vi "HFRR ADV v01.vi"() -> ()   [LabVIEW 2025] (continued)
              tunnel: w635 -> [w689 _]
              frame False {
                n427 = Equal?(x=w692, y="\"line\"") -> (x = y?=w694:bool)
                n428 = case shown="True" w694 {
                  tunnel: w693 -> [_ w709]
                  tunnel: w691 -> [w696 w708]
                  tunnel: [w696 w706] -> w690
                  tunnel: w689 -> [_ w705]
                  frame False {
                  }
                  frame True {
                    w704 = 0.0 ("Major Axis")
                    n429 = Match Pattern(string=w709, regular expression="\"length_px\":") -> (after substring=w707:string)  [unwired: 1 in, 3 out]
                    n430 = property on="Major Axis" class="DigNum (strict)"("Caption.Text"="") -> ()  [unwired: 2 in, 2 out]
                    n431 = property on="Minor Axis" class="DigNum (strict)"("Caption.Text"="") -> ()  [unwired: 2 in, 2 out]
                    n432 = property on="Average" class="DigNum (strict)"("Caption.Text"="Line") -> ()  [unwired: 2 in, 2 out]
                    n433 = Fract/Exp String To Number(string=w707, default (0 dbl)=0.0 ("default (0 DBL)")) -> (number=w703:dbl)  [unwired: 2 in, 1 out]
                    "Pixel Value" <- w703
                    n434 = Multiply(x=w703, y=w705) -> (x*y=w716:dbl)
                    n435 = Multiply(x=w716, y=1000.0) -> (x*y=w699:dbl)
                    n436 = Divide(x=w699, y=1000.0) -> (x/y=w702:dbl)
                    n437 = local write "Measurment (mm)"(w702) -> ()
                    n438 = Bundle By Name(cluster=w708, "average"=w699) -> (w706:cluster{"major":dbl, "minor":dbl, "average":dbl})
                    n439 = Number To Fractional String(number=w699, precision (6)=i16 1) -> (F-format string=w698:string)  [unwired: 2 in]
                    n440 = local write "Minor Axis"(w704) -> ()
                    n441 = local write "Major Axis"(w704) -> ()
                    n442 = Fract/Exp String To Number(string=w698) -> (number=w697:dbl)  [unwired: 3 in, 1 out]
                    n443 = local write "Average"(w697) -> ()
                  }
                }
              }
              frame True {
                w736 = 1000.0 ("y")
                w742 = 0.0 ("default (0 DBL)")
                n444 = Match Pattern(string=w748, regular expression=" \"width_px\":") -> (after substring=w746:string)  [unwired: 1 in, 3 out]
                n445 = Match Pattern(string=w746, regular expression="\"height_px\":") -> (before substring=w744:string, after substring=w743:string)  [unwired: 1 in, 2 out]
                n446 = Fract/Exp String To Number(string=w744, default (0 dbl)=w742) -> (number=w741:dbl)  [unwired: 2 in, 1 out]
                n447 = Fract/Exp String To Number(string=w743, default (0 dbl)=w742) -> (number=w740:dbl)  [unwired: 2 in, 1 out]
                n448 = Multiply(x=w741, y=w739) -> (x*y=w738:dbl)
                n449 = Multiply(x=w740, y=w739) -> (x*y=w737:dbl)
                n450 = Multiply(x=w738, y=w736) -> (x*y=w722:dbl)
                n451 = Multiply(x=w737, y=w736) -> (x*y=w720:dbl)
                n452 = Add(x=w722, y=w720) -> (x+y=w734:dbl)
                n453 = property on="Major Axis" class="DigNum (strict)"("Caption.Text"="Major Axis") -> ()  [unwired: 2 in, 2 out]
                n454 = property on="Minor Axis" class="DigNum (strict)"("Caption.Text"="Minor Axis") -> ()  [unwired: 2 in, 2 out]
                n455 = property on="Average" class="DigNum (strict)"("Caption.Text"="Average") -> ()  [unwired: 2 in, 2 out]
                n456 = Divide(x=w734, y=2.0) -> (x/y=w718:dbl)
                n457 = Bundle By Name(cluster=w735, "major"=w722, "minor"=w720, "average"=w718) -> (w732:cluster{"major":dbl, "minor":dbl, "average":dbl})
                n458 = Number To Fractional String(number=w720, precision (6)=i16 1) -> (F-format string=w727:string)  [unwired: 2 in]
                n459 = Number To Fractional String(number=w718, precision (6)=i16 1) -> (F-format string=w728:string)  [unwired: 2 in]
                n460 = Number To Fractional String(number=w722, precision (6)=i16 1) -> (F-format string=w726:string)  [unwired: 2 in]
                n461 = Fract/Exp String To Number(string=w727) -> (number=w719:dbl)  [unwired: 3 in, 1 out]
                n462 = Fract/Exp String To Number(string=w728) -> (number=w717:dbl)  [unwired: 3 in, 1 out]
                n463 = Fract/Exp String To Number(string=w726) -> (number=w721:dbl)  [unwired: 3 in, 1 out]
                n464 = local write "Major Axis"(w721) -> ()
                n465 = local write "Average"(w717) -> ()
                n466 = local write "Minor Axis"(w719) -> ()
              }
            }
            n467 = case shown="\"Measrument\", Default" w631 {
              tunnel: w634 -> [w661 _]
              tunnel: w633 -> [w660 _]
              tunnel: [w657 w686] -> w632
              tunnel: w630 -> [w659 w686]
              tunnel: w629 -> [w658 _]
              tunnel: w626 -> [w656 _]
              frame "Measrument", Default {
                n468 = stacked-sequence {
                  tunnel: w661 -> [w679 _]
                  tunnel: w660 -> [w677 _]
                  tunnel: w659 -> [w675 _]
                  tunnel: w658 -> [w674 _]
                  tunnel: [w669 _] -> w657
                  tunnel: w656 -> [w662 _]
                  frame #0 {
                    n469 = call "IMAGE ANALYSIS.vi"("Enum"=POST_ANALYSIS_ENUM."SAVE IMAGE", "error in"=w675, "IMAGE FILE PATH"=w674) -> ("error out"=w673:errorcluster)  [unwired: 7 in, 1 out]
                    n470 = call "Stall Data Flow.vim"("value in"=w673, "milliseconds to wait"=u32 1000) -> ("value out"=w664:errorcluster)  [unwired: 1 out]
                    n471 = local read "Test File List :"() -> (w681:string)
                    n472 = call "IMAGE ANALYSIS.vi"("Enum"=POST_ANALYSIS_ENUM."MINIMIZE UI", "error in"=w664) -> ("error out"=w671:errorcluster)  [unwired: 8 in, 1 out]
                    n473 = Bundle By Name(cluster=T20 {"File Name"="", "Test Method"="", "Operator"="", "Fuel Description"="", "Date and time"=""} ("Main Ref"), "Test Method"=w662, "File Name"=w681) -> (w682:T20)
                    n474 = call "Stall Data Flow.vim"("value in"=w671, "milliseconds to wait"=u32 1500) -> ("value out"=w666:errorcluster)  [unwired: 1 out]
                    n475 = call "duf file read.vi"("error in (no error)"=w666, "Main Ref"=w682) -> ("error out"=w680:errorcluster, "Main Ref 2"=w678:T20)  [unwired: 8 in]
                    n476 = call "DETECTION REPORT for manual.vi"("error in (no error)"=w680, "return value 3"=w677, "Image File Path"=w679, "Main Ref"=w678) -> ("error out"=w676:errorcluster)  [unwired: 7 in]
                    n477 = call <vilib>:"Clear Errors.vi"("error in (no error)"=w676) -> ("error out"=w667:errorcluster)  [unwired: 5 in, 1 out]
                    n478 = call "IMAGE ANALYSIS.vi"("Enum"=POST_ANALYSIS_ENUM."MINIMIZE UI", "error in"=w667) -> ("error out"=w669:errorcluster)  [unwired: 8 in, 1 out]
                  }
                  frame #1 {
                    n479 = local write "Main Tab"(T2."HOME" ("Main Tab")) -> ()
                    n480 = local write "Main Dashboard Buttons"(T1."Home" ("Main Dashboard Buttons")) -> ()
                  }
                }
              }
              frame "Calibrate" {
              }
            }
          }
          frame #2 {
            n481 = Not(x=w751) -> (.not. x?=w750:bool)
            n482 = local write "Confirm Measrurement"(w750) -> ()
            n483 = local read "Calibration Tab"() -> (w749:enum32{"Measrument", "Calibrate"})
            n484 = case shown="\"Measrument\", Default" w749 {
              frame "Measrument", Default {
                n485 = local write "Main Tab"(T2."HOME" ("Main Tab")) -> ()
              }
              frame "Calibrate" {
              }
            }
          }
        }
      }
    }
    n486 = local read "Humidity"() -> (w494:bool)
    n487 = local read "Save Change"() -> (w499:bool)
    n488 = local read "Calibrate"() -> (w500:bool)
    n489 = local read "Auto Start Test"() -> (w495:bool)
    n490 = case shown="True" w500 {
      selector: w500 -> [_ w607]
      frame False {
      }
      frame True {
        n491 = Not(x=w607) -> (.not. x?=w606:bool)
        n492 = local write "Calibrate"(w606) -> ()
        n493 = local write "Calibration Tab"(enum32{"Measrument", "Calibrate"}."Calibrate" ("Calibration Tab")) -> ()
      }
    }
    n494 = case shown="True" w499 {
      selector: w499 -> [_ w551]
      frame False {
      }
      frame True {
        n495 = stacked-sequence {
          tunnel: w551 -> [_ _ _ _ w605]
          frame #0 {
            n496 = call "IMAGE ANALYSIS.vi"("Enum"=POST_ANALYSIS_ENUM."HIDE UI") -> ()  [unwired: 9 in, 2 out]
          }
          frame #1 {
            n497 = local read "100x gain"() -> (w553:dbl)
            n498 = local read "10x Gain"() -> (w554:dbl)
            n499 = local read "5x Gain"() -> (w555:dbl)
            n500 = Number To Fractional String(number=w554, width (-)=i16 4, precision (6)=i16 7) -> (F-format string=w576:string)  [unwired: 1 in]
            n501 = Number To Fractional String(number=0.0, width (-)=i16 4, precision (6)=i16 7) -> (F-format string=w571:string)  [unwired: 1 in]
            n502 = Number To Fractional String(number=w553, width (-)=i16 4, precision (6)=i16 7) -> (F-format string=w559:string)  [unwired: 1 in]
            n503 = Number To Fractional String(number=w555, width (-)=i16 10 ("precision (6)"), precision (6)=i16 7) -> (F-format string=w585:string)  [unwired: 1 in]
            n504 = Concatenate Strings("[CH1]" ("string"), w585, " - 5x Gain" ("string"), "\r") -> (w575:string)
            n505 = Concatenate Strings("[CH2]" ("string"), w576, " - 10x Gain" ("string"), "\r") -> (w574:string)
            n506 = Concatenate Strings("[CH3]" ("string"), w571, " - 20x Gain" ("string"), "\r") -> (w565:string)
            n507 = Concatenate Strings("[CH4]" ("string"), w559, " - 100x Gain" ("string"), "\r") -> (w558:string)
            n508 = String To Path(string="C:\\LAB-IQ\\Image Calibrate v01.dcf") -> (path=w588:path)
            n509 = Concatenate Strings(w575, w574, w565, w558) -> (w573:string)
            n510 = call <vilib>:"Write Characters To File.vi"("append to file? (new file:F)"=FALSE, "character string"=w573, "file path (dialog if empty)"=w588) -> ()  [unwired: 2 in, 1 out]
          }
          frame #2 {
            n511 = String To Path(string="C:\\LAB-IQ\\Image Calibrate v01.dcf") -> (path=w591:path)
            n512 = Open/Create/Replace File ("Open File")(file path (use dialog)=w591) -> (refnum out=w592:refnum<file>)  [unwired: 5 in, 2 out]
            n513 = for {
              N: 4 -> [_]
              tunnel: w592 -> [w598]
              i -> [w594]
              n514 = Read from Text File ("Read File")(file (use dialog)=w598) -> (text=w599:string)  [unwired: 3 in, 3 out]
              n515 = String Subset(string=w599, offset (0)=6, length (rest)=10 ("length (rest)")) -> (substring=w595:string)
              n516 = Fract/Exp String To Number(string=w595) -> (number=w593:dbl)  [unwired: 3 in, 1 out]
              n517 = case shown="3" w594 {
                tunnel: w593 -> [w600 w601 _ w602 _]
                frame 0 {
                  n518 = local write "5x Gain"(w600) -> ()
                }
                frame 1 {
                  n519 = local write "10x Gain"(w601) -> ()
                }
                frame 2 {
                }
                frame 3 {
                  n520 = local write "100x gain"(w602) -> ()
                }
                frame 4, Default {
                }
              }
            }
          }
          frame #3 {
            n521 = call "IMAGE ANALYSIS.vi"("Enum"=POST_ANALYSIS_ENUM."SHOW UI") -> ()  [unwired: 9 in, 2 out]
          }
          frame #4 {
            n522 = Not(x=w605) -> (.not. x?=w604:bool)
            n523 = local write "Save Change"(w604) -> ()
          }
        }
      }
    }
    n524 = case shown="False" w495 {
      tunnel: w494 -> [w521 _]
      frame False {
        n525 = case shown="True" w521 {
          frame False {
          }
          frame True {
            n526 = local read "Set Humidity:"() -> (w525:dbl)
            n527 = local read "Set Humidity:"() -> (w528:dbl)
            n528 = local read "Humidity ( %RH )"() -> (w529:dbl)
            n529 = Subtract(x=w525, y=2.0) -> (x-y=w523:dbl)
            n530 = Add(x=w528, y=2.0) -> (x+y=w524:dbl)
            n531 = In Range and Coerce(upper limit=w524, x=w529, lower limit=w523) -> (In Range?=w522:bool)  [unwired: 1 out]
            n532 = case shown="True" w522 {
              frame False {
              }
              frame True {
                n533 = case shown="False" "Manual Humididty Reached" {
                  selector: "Manual Humididty Reached" -> [_ w532]
                  frame False {
                  }
                  frame True {
                    n534 = Not(x=w532) -> (.not. x?=w531:bool)
                    n535 = local write "Manual Humididty Reached"(w531) -> ()
                    n536 = local read "EVENT LOG"() -> (w534:string)
                    n537 = call "Event Log.vi"("Content"="Target Humidity reached", "EVENT LOG"=w534) -> ("EVENT LOG"=w533:string)  [unwired: 8 in, 1 out]
                    n538 = local write "EVENT LOG"(w533) -> ()
                  }
                }
              }
            }
          }
        }
      }
      frame True {
        n539 = local write "Manual Humididty Reached"(TRUE ("Manual Humididty Reached")) -> ()
      }
    }
    n540 = local read "Cap Live Image"() -> (w515:bool)
    n541 = local read "SCAR MEASURMENT"() -> (w518:enum32{"Auto Scar", "Manual Scar"})
    n542 = Wait (ms)(milliseconds to wait=u32 250) -> ()  [unwired: 1 out]
    n543 = Equal?(x=w518, y=enum32{"Auto Scar", "Manual Scar"}."Manual Scar" ("SCAR MEASURMENT")) -> (x = y?=w516:bool)
    n544 = And(x=w516, y=w515) -> (x .and. y?=w514:bool)
    n545 = case shown="True" w514 {
      selector: w514 -> [_ w830]
      frame False {
      }
      frame True {
        n546 = stacked-sequence {
          tunnel: [_ _ _ w845 _] -> _
          tunnel: w830 -> [_ _ _ _ w851]
          frame #0 {
            w831 = 0.0
            n547 = local write "Major Axis"(w831) -> ()
            n548 = local write "Minor Axis"(w831) -> ()
            n549 = local write "Average"(w831) -> ()
          }
          frame #1 {
            n550 = call "CAMERA LIVE FEED FGV.vi"("Enum - Menu"=CAMERA_LIVE_FEED_ENUM."CAMERA MINIMIZE") -> ()  [unwired: 9 in, 2 out]
          }
          frame #2 {
            n551 = local read "FILE 3"() -> (w839:string)
            n552 = call <vilib>:"Trim Whitespace.vi"("string"="C:\\LAB-IQ\\images\\") -> ("trimmed string"=w841:string)  [unwired: 1 in]
            n553 = String To Path(string=w841) -> (path=w840:path)
            n554 = Concatenate Strings(w839, ".png" ("string")) -> (w838:string)
            n555 = Build Path(base path=w840, name or relative path=w838) -> (appended path=w836:path)
            n556 = Path To String(path=w836) -> (string=w835:string)
            n557 = call "CAMERA LIVE FEED FGV.vi"("Enum - Menu"=CAMERA_LIVE_FEED_ENUM."CAMERA SAVE", "Image Path"=w835) -> ("error out"=w833:errorcluster)  [unwired: 8 in, 1 out]
            n558 = case shown="No Error" w833 {
              frame No Error {
                n559 = One Button Dialog(message="Image saved successfully") -> ()  [unwired: 1 in, 1 out]
              }
              frame Error {
              }
            }
          }
          frame #3 {
            n560 = call "LIST FILE NAMES.vi"() -> ("error out"=w847:errorcluster, "filenames"=w844:string[])  [unwired: 10 in]
            n561 = call "IMAGE ANALYSIS.vi"("Enum"=POST_ANALYSIS_ENUM."SHOW UI", "error in"=w847) -> ("error out"=w845:errorcluster)  [unwired: 8 in, 1 out]
            n562 = property on="Test File List :" class="CmbBox"("Strings[]"=w844) -> ()  [unwired: 2 in, 2 out]
          }
          frame #4 {
            (unwired) T21."Report" ("Main Dashboard Buttons")
            n563 = Not(x=w851) -> (.not. x?=w850:bool)
            n564 = local write "Zoom Factore"(0.0 ("Zoom Factore")) -> ()
            n565 = local write "Cap Live Image"(w850) -> ()
            n566 = local write "Main Tab"(T2."Adv Scar Report" ("Main Tab")) -> ()
            n567 = property on="Cap Live Image" class="Bool (strict)"("BoolText.Text"="Capture Image" ("Boolean Text.Text")) -> ()  [unwired: 2 in, 2 out]
            n568 = local write "Main Dashboard Buttons"(T1."Report" ("Main Dashboard Buttons")) -> ()
          }
        }
      }
    }
    n569 = local read "change Gain"() -> (w498:bool)
    n570 = local read "Back Square"() -> (w497:bool)
    n571 = case shown="True" w498 {
      selector: w498 -> [_ w542]
      frame False {
      }
      frame True {
        n572 = stacked-sequence {
          tunnel: w542 -> [_ w550]
          frame #0 {
            n573 = local read "Actual (µm)"() -> (w546:dbl)
            n574 = local read "Pixel Value"() -> (w545:dbl)
            n575 = local read "Magnification :"() -> (w544:string)
            n576 = Divide(x=w546, y=w545) -> (x/y=w543:dbl)
            n577 = case shown="\"10x\"" w544 {
              tunnel: w543 -> [w547 w548]
              frame "10x" {
                n578 = local write "10x Gain"(w547) -> ()
              }
              frame "5x", Default {
                n579 = local write "5x Gain"(w548) -> ()
              }
            }
          }
          frame #1 {
            n580 = Not(x=w550) -> (.not. x?=w549:bool)
            n581 = local write "change Gain"(w549) -> ()
          }
        }
      }
    }
    n582 = case shown="True" w497 {
      selector: w497 -> [_ w540]
      frame False {
      }
      frame True {
        n583 = Not(x=w540) -> (.not. x?=w539:bool)
        n584 = local write "Back Square"(w539) -> ()
        n585 = local write "Calibration Tab"(enum32{"Measrument", "Calibrate"}."Measrument" ("Calibration Tab")) -> ()
      }
    }
    n586 = local read "Rectangle Tool"() -> (w509:bool)
    n587 = local read "Clear ROI Tool"() -> (w508:bool)
    n588 = local read "Open Image"() -> (w513:bool)
    n589 = local read "line tool"() -> (w510:bool)
    n590 = local read "OUT"() -> (w511:bool)
    n591 = local read "In"() -> (w512:bool)
    n592 = case shown="True" w513 {
      selector: w513 -> [_ w818]
      tunnel: [w814 w820] -> _
      tunnel: w503 -> [w814 w819]
      frame False {
      }
      frame True {
        n593 = Not(x=w818) -> (.not. x?=w817:bool)
        n594 = local write "Open Image"(w817) -> ()
        n595 = call "IMAGE ANALYSIS.vi"("Enum"=POST_ANALYSIS_ENUM."HIDE UI", "error in"=w819) -> ("error out"=w827:errorcluster)  [unwired: 8 in, 1 out]
        n596 = call "File Dialog"("start path"=path "C:/LAB-IQ/images", "error in"=w827) -> ("selected path"=w816:path, "error out"=w825:errorcluster)  [unwired: 10 in, 2 out]
        "Image path  2" <- w816
        n597 = call <vilib>:"Clear Errors.vi"("error in (no error)"=w825) -> ("error out"=w824:errorcluster)  [unwired: 5 in, 1 out]
        n598 = call "IMAGE ANALYSIS.vi"("Enum"=POST_ANALYSIS_ENUM."OPEN FILE", "error in"=w824, "File Path"=w816) -> ("error out"=w823:errorcluster)  [unwired: 7 in, 1 out]
        n599 = call <vilib>:"Clear Errors.vi"("error in (no error)"=w823) -> ("error out"=w822:errorcluster)  [unwired: 5 in, 1 out]
        n600 = call "IMAGE ANALYSIS.vi"("Enum"=POST_ANALYSIS_ENUM."SHOW UI", "error in"=w822) -> ("error out"=w820:errorcluster)  [unwired: 8 in, 1 out]
        n601 = local write "Zoom Factore"(100.0 ("Zoom Factore")) -> ()
      }
    }
    n602 = case shown="True" w511 {
      selector: w511 -> [_ w799]
      tunnel: w503 -> [w796 w804]
      tunnel: [w796 w798] -> _
      frame False {
      }
      frame True {
        n603 = Not(x=w799) -> (.not. x?=w797:bool)
        n604 = local read "Zoom Factore"() -> (w802:dbl)
        n605 = local write "OUT"(w797) -> ()
        n606 = call "IMAGE ANALYSIS.vi"("Enum"=POST_ANALYSIS_ENUM."ZOOM OUT", "error in"=w804) -> ("error out"=w798:errorcluster)  [unwired: 8 in, 1 out]
        n607 = Divide(x=w802, y=1.2) -> (x/y=w800:dbl)
        n608 = local write "Zoom Factore"(w800) -> ()
      }
    }
    n609 = case shown="True" w512 {
      selector: w512 -> [_ w808]
      tunnel: w503 -> [w805 w813]
      tunnel: [w805 w806] -> _
      frame False {
      }
      frame True {
        n610 = Not(x=w808) -> (.not. x?=w807:bool)
        n611 = local read "Zoom Factore"() -> (w811:dbl)
        n612 = local write "In"(w807) -> ()
        n613 = call "IMAGE ANALYSIS.vi"("Enum"=POST_ANALYSIS_ENUM."ZOOM IN", "error in"=w813) -> ("error out"=w806:errorcluster)  [unwired: 8 in, 1 out]
        n614 = Multiply(x=w811, y=1.2) -> (x*y=w809:dbl)
        n615 = local write "Zoom Factore"(w809) -> ()
      }
    }
    n616 = case shown="True" w508 {
      selector: w508 -> [_ w780]
      tunnel: w503 -> [w778 w782]
      tunnel: [w778 w781] -> _
      frame False {
      }
      frame True {
        n617 = Not(x=w780) -> (.not. x?=w779:bool)
        n618 = local write "Clear ROI Tool"(w779) -> ()
        n619 = call "IMAGE ANALYSIS.vi"("Enum"=POST_ANALYSIS_ENUM."CLEAR ROI", "error in"=w782) -> ("error out"=w781:errorcluster)  [unwired: 8 in, 1 out]
      }
    }
    n620 = case shown="True" w510 {
      selector: w510 -> [_ w792]
      tunnel: w503 -> [w790 w795]
      tunnel: [w790 w793] -> _
      frame False {
      }
      frame True {
        n621 = Not(x=w792) -> (.not. x?=w791:bool)
        n622 = local write "line tool"(w791) -> ()
        n623 = call "IMAGE ANALYSIS.vi"("Enum"=POST_ANALYSIS_ENUM."DRAW LINE", "error in"=w795) -> ("error out"=w793:errorcluster)  [unwired: 8 in, 1 out]
      }
    }
    n624 = case shown="True" w509 {
      selector: w509 -> [_ w786]
      tunnel: w503 -> [w784 w788]
      tunnel: [w784 w787] -> _
      frame False {
      }
      frame True {
        n625 = Not(x=w786) -> (.not. x?=w785:bool)
        n626 = local write "Rectangle Tool"(w785) -> ()
        n627 = call "IMAGE ANALYSIS.vi"("Enum"=POST_ANALYSIS_ENUM."DRAW REC", "error in"=w788) -> ("error out"=w787:errorcluster)  [unwired: 8 in, 1 out]
      }
    }
    n628 = local read "SCAR MEASURMENT"() -> (w496:enum32{"Auto Scar", "Manual Scar"})
    n629 = local read "Fit to Screen Tool"() -> (w505:bool)
    n630 = local read "Resize Tool"() -> (w504:bool)
    n631 = case shown="\"Manual Scar\", Default" w496 {
      frame "Auto Scar" {
        n632 = property on="Cap Live Image" class="Bool (strict)"("BoolText.Text"="Report" ("Boolean Text.Text")) -> ()  [unwired: 2 in, 2 out]
      }
      frame "Manual Scar", Default {
        n633 = property on="Cap Live Image" class="Bool (strict)"("BoolText.Text"="Save Image" ("Boolean Text.Text")) -> ()  [unwired: 2 in, 2 out]
      }
    }
    n634 = local read "ROI Color Tool"() -> (w506:bool)
    n635 = local read "Pan Tool"() -> (w507:bool)
    n636 = case shown="True" w507 {
      selector: w507 -> [_ w774]
      tunnel: w503 -> [w772 w776]
      tunnel: [w772 w775] -> _
      frame False {
      }
      frame True {
        n637 = Not(x=w774) -> (.not. x?=w773:bool)
        n638 = call "IMAGE ANALYSIS.vi"("Enum"=POST_ANALYSIS_ENUM."PAN", "error in"=w776) -> ("error out"=w775:errorcluster)  [unwired: 8 in, 1 out]
        n639 = local write "Pan Tool"(w773) -> ()
      }
    }
    n640 = case shown="True" w504 {
      selector: w504 -> [_ w758]
      tunnel: w503 -> [w753 w755]
      tunnel: [w753 w754] -> _
      frame False {
      }
      frame True {
        n641 = Not(x=w758) -> (.not. x?=w757:bool)
        n642 = local write "Resize Tool"(w757) -> ()
        n643 = call "IMAGE ANALYSIS.vi"("Enum"=POST_ANALYSIS_ENUM."RESIZE MODE", "error in"=w755) -> ("error out"=w754:errorcluster)  [unwired: 8 in, 1 out]
      }
    }
    n644 = case shown="True" w505 {
      selector: w505 -> [_ w763]
      tunnel: [w759 w764] -> _
      tunnel: w503 -> [w759 w762]
      frame False {
      }
      frame True {
        n645 = Not(x=w763) -> (.not. x?=w761:bool)
        n646 = local write "Zoom Factore"(100.0 ("Zoom Factore")) -> ()
        n647 = local write "Fit to Screen Tool"(w761) -> ()
        n648 = call "IMAGE ANALYSIS.vi"("Enum"=POST_ANALYSIS_ENUM."FIT", "error in"=w762) -> ("error out"=w764:errorcluster)  [unwired: 8 in, 1 out]
      }
    }
    n649 = case shown="True" w506 {
      selector: w506 -> [_ w769]
      tunnel: [w766 w770] -> _
      tunnel: w503 -> [w766 w767]
      frame False {
      }
      frame True {
        n650 = Not(x=w769) -> (.not. x?=w768:bool)
        n651 = local write "ROI Color Tool"(w768) -> ()
        n652 = call "IMAGE ANALYSIS.vi"("Enum"=POST_ANALYSIS_ENUM."SET ROI COLOR", "error in"=w767) -> ("error out"=w770:errorcluster)  [unwired: 8 in, 1 out]
      }
    }
    n653 = local read "Quit"() -> (w520:bool)
  }
  n654 = while {
    stop <- w854 stop-if-true
    n655 = local read "Image Path"() -> (w857:path)
    n656 = local read "Print 3"() -> (w860:bool)
    n657 = Equal?(x=w857, y=path "") -> (x = y?=w856:bool)
    n658 = Not(x=w856) -> (.not. x?=w855:bool)
    n659 = property on="Print 3" class="Bool (strict)"("Visible"=w855) -> ()  [unwired: 2 in, 2 out]
    n660 = case shown="True" w860 {
      frame False {
        n661 = local write "Rd"(TRUE ("Boolean 7")) -> ()
      }
      frame True {
        n662 = flat-sequence {
          tunnel: [w900] -> w868
          tunnel: [w887] -> w866
          tunnel: [w897] -> w862
          tunnel: w868 -> [w909]
          tunnel: [w909] -> w867
          tunnel: w866 -> [w908]
          tunnel: [w908] -> w865
          tunnel: [w906] -> w864
          tunnel: [w905] -> w863
          tunnel: w862 -> [w905]
          tunnel: w867 -> [w911]
          tunnel: w865 -> [w912]
          tunnel: w864 -> [_]
          tunnel: w863 -> [w910]
          frame #0 {
            n663 = case shown="True" "Rd" {
              frame False {
              }
              frame True {
                n664 = while {
                  tunnel: "abcdefABCDEF" ("string 2") -> [w879]
                  shift-right: [w877] -> w871
                  shift-left: "" -> [w876]
                  i -> [w886]
                  stop <- w885 stop-if-true
                  n665 = Random Number (0-1)() -> (number: 0 to 1=w880:dbl)
                  n666 = Multiply(x=w880, y=62.0) -> (x*y=w882:dbl)
                  n667 = Decrement(x="Length 2") -> (x-1=w875:i16)
                  n668 = To Word Integer(number=w882) -> (16bit integer=w883:i16)
                  n669 = String Subset(string=w879, offset (0)=w883, length (rest)=1 ("length (rest)")) -> (substring=w878:string)
                  n670 = Greater Or Equal?(x=w886, y=w875) -> (x >= y?=w885:bool)
                  n671 = Concatenate Strings(w878, w876) -> (w877:string)
                }
                "String 10" <- w871
                n672 = local write "Rd"(FALSE ("Boolean 7")) -> ()
              }
            }
          }
          frame #1 {
            w898 = "_resized.jpg" ("command line")
            (unwired) ".jpg -resize 320x240 " ("string")
            (unwired) "Choose an Image File" ("prompt")
            # "-resize 1798x425"
            n673 = local read "Image Path"() -> (w892:path)
            n674 = Strip Path(path=w892) -> (stripped path=w887:path, name=w888:string)
            n675 = Match Pattern(string=w888, regular expression=".jpg") -> (before substring=→"before substring 2":string, after substring=→"after substring":string)  [unwired: 1 in, 2 out]
            n676 = Match Pattern(string=w888, regular expression="\\") -> (before substring=w894:string)  [unwired: 1 in, 3 out]
            n677 = Match Pattern(string=w894, regular expression=".jpg") -> (before substring=w893:string)  [unwired: 1 in, 3 out]
            n678 = Concatenate Strings("cmd /c convert " ("string"), w893, ".jpg -resize 320x240  " ("command line"), w893, w898) -> (w901:string)
            n679 = call <vilib>:"System Exec.vi"("run minimized? (F)"=TRUE, "wait until completion? (T)"=TRUE, "working directory"=w887, "command line"=w901) -> ("error out"=w900:errorcluster)  [unwired: 4 in, 3 out]
            "error out 2" <- w900
            n680 = Concatenate Strings(w893, w898) -> (w897:string)
          }
          frame #2 {
            n681 = Wait (ms)(milliseconds to wait=u32 2000 ("millisecond timer value")) -> (millisecond timer value=w906:u32)
          }
          frame #3 {
            n682 = case shown="No Error" w911 {
              tunnel: w912 -> [w915 _]
              tunnel: w910 -> [w913 _]
              frame No Error {
                (unwired) ".jpg" ("string")
                n683 = Path To String(path=w915) -> (string=w919:string)
                n684 = Concatenate Strings(w919, "\\" ("string"), w913) -> (w918:string)
                n685 = String To Path(string=w918) -> (path=w917:path)
                n686 = call <vilib>:"Read JPEG File.vi"("path to JPEG file"=w917) -> ("image data"=w921:T13)  [unwired: 8 in, 2 out]
                "image data" <- w921
                n687 = local write "Print 3"(FALSE ("Print 2")) -> ()
                n688 = call <vilib>:"Draw Flattened Pixmap.vi"("image data"=w921) -> ("new picture"=→"new picture":picture)  [unwired: 8 in]
              }
              frame Error {
              }
            }
          }
        }
      }
    }
    n689 = Wait (ms)(milliseconds to wait=u32 20 ("millisecond timer value")) -> ()  [unwired: 1 out]
    n690 = local read "Quit"() -> (w854:bool)
  }
  n691 = property on="Service Password Log" class="Str"("Visible"=w9) -> ()  [unwired: 2 in, 2 out]
  n692 = property on="Password 3" class="Clust (strict)"("Visible"=w9) -> ()  [unwired: 2 in, 2 out]
  n693 = while {
    tunnel: w30 -> [_]
    tunnel: w13 -> [_]
    stop <- w952 stop-if-true
    # "New Adv Logics"
    n694 = local read "Main Tab"() -> (w931:T2)
    n695 = local read "Main Tab"() -> (w950:T2)
    n696 = local read "Sign In"() -> (w949:bool)
    n697 = case shown="\"Adv Scar\"" w931 {
      frame "HOME", Default {
        n698 = local read "LIVE FEED MIN TEMP"() -> (w1079:bool)
        n699 = local write "LIVE FEED MAX TEMP"(TRUE ("LIVE FEED MAX TEMP")) -> ()
        n700 = local read "CAMERA ROI MIN TEMP"() -> (w1077:bool)
        n701 = case shown="True" w1079 {
          selector: w1079 -> [_ w1086]
          frame False {
          }
          frame True {
            n702 = Not(x=w1086) -> (.not. x?=w1085:bool)
            n703 = local write "LIVE FEED MIN TEMP"(w1085) -> ()
            n704 = call "CAMERA LIVE FEED FGV.vi"("Enum - Menu"=CAMERA_LIVE_FEED_ENUM."CAMERA MINIMIZE") -> ()  [unwired: 9 in, 2 out]
          }
        }
        n705 = case shown="True" w1077 {
          selector: w1077 -> [_ w1083]
          frame False {
          }
          frame True {
            n706 = Not(x=w1083) -> (.not. x?=w1082:bool)
            n707 = local write "CAMERA ROI MIN TEMP"(w1082) -> ()
            n708 = call "IMAGE ANALYSIS.vi"("Enum"=POST_ANALYSIS_ENUM."MINIMIZE UI") -> ()  [unwired: 9 in, 2 out]
          }
        }
        n709 = local write "CAMERA ROI MAX TEMP"(TRUE ("CAMERA ROI MAX TEMP")) -> ()
      }
      frame "Test Setup" {
        n710 = local read "LIVE FEED MIN TEMP"() -> (w1089:bool)
        n711 = local read "CAMERA ROI MIN TEMP"() -> (w1087:bool)
        n712 = local write "LIVE FEED MAX TEMP"(TRUE ("LIVE FEED MAX TEMP")) -> ()
        n713 = case shown="True" w1089 {
          selector: w1089 -> [_ w1096]
          frame False {
          }
          frame True {
            n714 = Not(x=w1096) -> (.not. x?=w1095:bool)
            n715 = local write "LIVE FEED MIN TEMP"(w1095) -> ()
            n716 = call "CAMERA LIVE FEED FGV.vi"("Enum - Menu"=CAMERA_LIVE_FEED_ENUM."CAMERA MINIMIZE") -> ()  [unwired: 9 in, 2 out]
          }
        }
        n717 = case shown="True" w1087 {
          selector: w1087 -> [_ w1093]
          frame False {
          }
          frame True {
            n718 = Not(x=w1093) -> (.not. x?=w1092:bool)
            n719 = local write "CAMERA ROI MIN TEMP"(w1092) -> ()
            n720 = call "IMAGE ANALYSIS.vi"("Enum"=POST_ANALYSIS_ENUM."MINIMIZE UI") -> ()  [unwired: 9 in, 2 out]
          }
        }
        n721 = local write "CAMERA ROI MAX TEMP"(TRUE ("CAMERA ROI MAX TEMP")) -> ()
      }
      frame "Acquire" {
        n722 = local read "LIVE FEED MIN TEMP"() -> (w1099:bool)
        n723 = local write "LIVE FEED MAX TEMP"(TRUE ("LIVE FEED MAX TEMP")) -> ()
        n724 = local read "CAMERA ROI MIN TEMP"() -> (w1097:bool)
        n725 = case shown="True" w1099 {
          selector: w1099 -> [_ w1106]
          frame False {
          }
          frame True {
            n726 = Not(x=w1106) -> (.not. x?=w1105:bool)
            n727 = local write "LIVE FEED MIN TEMP"(w1105) -> ()
            n728 = call "CAMERA LIVE FEED FGV.vi"("Enum - Menu"=CAMERA_LIVE_FEED_ENUM."CAMERA MINIMIZE") -> ()  [unwired: 9 in, 2 out]
          }
        }
        n729 = case shown="True" w1097 {
          selector: w1097 -> [_ w1103]
          frame False {
          }
          frame True {
            n730 = Not(x=w1103) -> (.not. x?=w1102:bool)
            n731 = local write "CAMERA ROI MIN TEMP"(w1102) -> ()
            n732 = call "IMAGE ANALYSIS.vi"("Enum"=POST_ANALYSIS_ENUM."MINIMIZE UI") -> ()  [unwired: 9 in, 2 out]
          }
        }
        n733 = local write "CAMERA ROI MAX TEMP"(TRUE ("CAMERA ROI MAX TEMP")) -> ()
      }
      frame "Adv Scar" {
        n734 = local read "CAMERA ROI MIN TEMP"() -> (w1107:bool)
        n735 = case shown="True" "LIVE FEED MAX TEMP" {
          selector: "LIVE FEED MAX TEMP" -> [_ w1128]
          frame False {
          }
          frame True {
            n736 = Not(x=w1128) -> (.not. x?=w1127:bool)
            n737 = local write "LIVE FEED MAX TEMP"(w1127) -> ()
            n738 = call "CAMERA LIVE FEED FGV.vi"("Enum - Menu"=CAMERA_LIVE_FEED_ENUM."CAMERA RESTORE") -> ("error out"=w1118:errorcluster)  [unwired: 9 in, 1 out]
            n739 = Type Cast(type=30, x=0) -> (*(type *) &x=w1122:i32)
            n740 = Add(x=w1122, y=48) -> (x+y=w1123:i32)
            n741 = call "CAMERA LIVE FEED FGV.vi"("Enum - Menu"=CAMERA_LIVE_FEED_ENUM."CAMERA MODE SET", "error in (no error)"=w1118, "CAMERA MODE"=w1123) -> ("error out"=w1115:errorcluster)  [unwired: 7 in, 1 out]
            n742 = call "CAMERA LIVE FEED FGV.vi"("Enum - Menu"=CAMERA_LIVE_FEED_ENUM."CAMERA GRAY", "error in (no error)"=w1115) -> ("error out"=w1114:errorcluster)  [unwired: 8 in, 1 out]
            n743 = call "LIST FILE NAMES.vi"("error in (no error)"=w1114) -> ("error out"=w1124:errorcluster, "filenames"=w1125:string[])  [unwired: 9 in]
            n744 = property on="FILE 3" class="CmbBox"(error in=w1124, "Strings[]"=w1125) -> ()  [unwired: 1 in, 2 out]
          }
        }
        n745 = case shown="True" w1107 {
          selector: w1107 -> [_ w1113]
          frame False {
          }
          frame True {
            n746 = Not(x=w1113) -> (.not. x?=w1112:bool)
            n747 = local write "CAMERA ROI MIN TEMP"(w1112) -> ()
            n748 = call "IMAGE ANALYSIS.vi"("Enum"=POST_ANALYSIS_ENUM."MINIMIZE UI") -> ()  [unwired: 9 in, 2 out]
          }
        }
        n749 = local write "CAMERA ROI MAX TEMP"(TRUE ("CAMERA ROI MAX TEMP")) -> ()
        "LIVE FEED MIN TEMP" <- TRUE ("LIVE FEED MIN TEMP")
      }
      frame "Adv Scar Report" {
        n750 = local read "CAMERA ROI MAX TEMP"() -> (w1129:bool)
        n751 = local read "LIVE FEED MIN TEMP"() -> (w1131:bool)
        n752 = local write "LIVE FEED MAX TEMP"(TRUE ("LIVE FEED MAX TEMP")) -> ()
        n753 = case shown="True" w1131 {
          selector: w1131 -> [_ w1140]
          frame False {
          }
          frame True {
            n754 = Not(x=w1140) -> (.not. x?=w1139:bool)
            n755 = local write "LIVE FEED MIN TEMP"(w1139) -> ()
            n756 = call "CAMERA LIVE FEED FGV.vi"("Enum - Menu"=CAMERA_LIVE_FEED_ENUM."CAMERA MINIMIZE") -> ()  [unwired: 9 in, 2 out]
          }
        }
        n757 = case shown="True" w1129 {
          selector: w1129 -> [_ w1137]
          frame False {
          }
          frame True {
            n758 = Not(x=w1137) -> (.not. x?=w1135:bool)
            n759 = local write "CAMERA ROI MAX TEMP"(w1135) -> ()
            n760 = call "IMAGE ANALYSIS.vi"("Enum"=POST_ANALYSIS_ENUM."SHOW UI") -> ("error out"=w1134:errorcluster)  [unwired: 9 in, 1 out]
            n761 = call "LIST FILE NAMES.vi"("error in (no error)"=w1134) -> ("filenames"=w1133:string[])  [unwired: 9 in, 1 out]
            n762 = property on="Test File List :" class="CmbBox"("Strings[]"=w1133) -> ()  [unwired: 2 in, 2 out]
          }
        }
        n763 = local write "CAMERA ROI MIN TEMP"(TRUE ("CAMERA ROI MIN TEMP")) -> ()
      }
      frame "Compare Files" {
        n764 = local read "LIVE FEED MIN TEMP"() -> (w1143:bool)
        n765 = local write "LIVE FEED MAX TEMP"(TRUE ("LIVE FEED MAX TEMP")) -> ()
        n766 = local read "CAMERA ROI MIN TEMP"() -> (w1141:bool)
        n767 = case shown="True" w1143 {
          selector: w1143 -> [_ w1150]
          frame False {
          }
          frame True {
            n768 = Not(x=w1150) -> (.not. x?=w1149:bool)
            n769 = local write "LIVE FEED MIN TEMP"(w1149) -> ()
            n770 = call "CAMERA LIVE FEED FGV.vi"("Enum - Menu"=CAMERA_LIVE_FEED_ENUM."CAMERA MINIMIZE") -> ()  [unwired: 9 in, 2 out]
          }
        }
        n771 = case shown="True" w1141 {
          selector: w1141 -> [_ w1147]
          frame False {
          }
          frame True {
            n772 = Not(x=w1147) -> (.not. x?=w1146:bool)
            n773 = local write "CAMERA ROI MIN TEMP"(w1146) -> ()
            n774 = call "IMAGE ANALYSIS.vi"("Enum"=POST_ANALYSIS_ENUM."MINIMIZE UI") -> ()  [unwired: 9 in, 2 out]
          }
        }
        n775 = local write "CAMERA ROI MAX TEMP"(TRUE ("CAMERA ROI MAX TEMP")) -> ()
      }
      frame "About" {
        n776 = local read "LIVE FEED MIN TEMP"() -> (w1153:bool)
        n777 = local write "LIVE FEED MAX TEMP"(TRUE ("LIVE FEED MAX TEMP")) -> ()
        n778 = local read "CAMERA ROI MIN TEMP"() -> (w1152:bool)
        n779 = case shown="True" w1153 {
          selector: w1153 -> [_ w1160]
          frame False {
          }
          frame True {
            n780 = Not(x=w1160) -> (.not. x?=w1159:bool)
            n781 = local write "LIVE FEED MIN TEMP"(w1159) -> ()
            n782 = call "CAMERA LIVE FEED FGV.vi"("Enum - Menu"=CAMERA_LIVE_FEED_ENUM."CAMERA MINIMIZE") -> ()  [unwired: 9 in, 2 out]
          }
        }
        n783 = case shown="True" w1152 {
          selector: w1152 -> [_ w1157]
          frame False {
          }
          frame True {
            n784 = Not(x=w1157) -> (.not. x?=w1156:bool)
            n785 = local write "CAMERA ROI MIN TEMP"(w1156) -> ()
            n786 = call "IMAGE ANALYSIS.vi"("Enum"=POST_ANALYSIS_ENUM."MINIMIZE UI") -> ()  [unwired: 9 in, 2 out]
          }
        }
        n787 = local write "CAMERA ROI MAX TEMP"(TRUE ("CAMERA ROI MIN TEMP")) -> ()
      }
      frame "Advance" {
        n788 = local read "LIVE FEED MIN TEMP"() -> (w1163:bool)
        n789 = local write "LIVE FEED MAX TEMP"(TRUE ("LIVE FEED MAX TEMP")) -> ()
        n790 = local read "CAMERA ROI MIN TEMP"() -> (w1161:bool)
        n791 = case shown="True" w1163 {
          selector: w1163 -> [_ w1170]
          frame False {
          }
          frame True {
            n792 = Not(x=w1170) -> (.not. x?=w1169:bool)
            n793 = local write "LIVE FEED MIN TEMP"(w1169) -> ()
            n794 = call "CAMERA LIVE FEED FGV.vi"("Enum - Menu"=CAMERA_LIVE_FEED_ENUM."CAMERA MINIMIZE") -> ()  [unwired: 9 in, 2 out]
          }
        }
        n795 = local write "CAMERA ROI MAX TEMP"(TRUE ("CAMERA ROI MAX TEMP")) -> ()
        n796 = case shown="True" w1161 {
          selector: w1161 -> [_ w1167]
          frame False {
          }
          frame True {
            n797 = Not(x=w1167) -> (.not. x?=w1166:bool)
            n798 = local write "CAMERA ROI MIN TEMP"(w1166) -> ()
            n799 = call "IMAGE ANALYSIS.vi"("Enum"=POST_ANALYSIS_ENUM."MINIMIZE UI") -> ()  [unwired: 9 in, 2 out]
          }
        }
      }
      frame "Mooha" {
        n800 = local read "LIVE FEED MIN TEMP"() -> (w1173:bool)
        n801 = local write "LIVE FEED MAX TEMP"(TRUE ("LIVE FEED MAX TEMP")) -> ()
        n802 = local read "CAMERA ROI MIN TEMP"() -> (w1171:bool)
        n803 = case shown="True" w1173 {
          selector: w1173 -> [_ w1180]
          frame False {
          }
          frame True {
            n804 = Not(x=w1180) -> (.not. x?=w1179:bool)
            n805 = local write "LIVE FEED MIN TEMP"(w1179) -> ()
            n806 = call "CAMERA LIVE FEED FGV.vi"("Enum - Menu"=CAMERA_LIVE_FEED_ENUM."CAMERA MINIMIZE") -> ()  [unwired: 9 in, 2 out]
          }
        }
        n807 = local write "CAMERA ROI MAX TEMP"(TRUE ("CAMERA ROI MAX TEMP")) -> ()
        n808 = case shown="True" w1171 {
          selector: w1171 -> [_ w1177]
          frame False {
          }
          frame True {
            n809 = Not(x=w1177) -> (.not. x?=w1176:bool)
            n810 = local write "CAMERA ROI MIN TEMP"(w1176) -> ()
            n811 = call "IMAGE ANALYSIS.vi"("Enum"=POST_ANALYSIS_ENUM."MINIMIZE UI") -> ()  [unwired: 9 in, 2 out]
          }
        }
      }
    }
    n812 = local read "Auto Start Test"() -> (w922:bool)
    n813 = case shown="True" "sign in temp" {
      frame False {
      }
      frame True {
        w959 = 1 ("y")
        n814 = local read "USERNAME"() -> (w965:string)
        n815 = local read "USER ID"() -> (w962:string)
        n816 = call <vilib>:"Trim Whitespace.vi"("string"=w965) -> ("trimmed string"=w964:string)  [unwired: 1 in]
        n817 = call <vilib>:"Trim Whitespace.vi"("string"=w962) -> ("trimmed string"=w963:string)  [unwired: 1 in]
        n818 = String Length(string=w964) -> (length=w961:i32)
        n819 = String Length(string=w963) -> (length=w960:i32)
        n820 = Greater?(x=w961, y=w959) -> (0:w958:bool)
        n821 = Greater?(x=w960, y=w959) -> (0:w957:bool)
        n822 = And(x=w958, y=w957) -> (x .and. y?=w956:bool)
        n823 = case shown="True" w956 {
          frame False {
            n824 = property on="Sign In" class="Bool (strict)"("DisabledEnum"=T15."Disabled" ("Disabled")) -> ()  [unwired: 2 in, 2 out]
          }
          frame True {
            n825 = property on="Sign In" class="Bool (strict)"("DisabledEnum"=T15."Enabled" ("Disabled")) -> ()  [unwired: 2 in, 2 out]
          }
        }
      }
    }
    n826 = local read "Air Temperature"() -> (w939:bool)
    n827 = local read "Coefficient Of Friction"() -> (w940:bool)
    n828 = case shown="False" w922 {
      frame False {
        n829 = local read "Auto stop temp"() -> (w953:bool)
        n830 = case shown="True" w953 {
          frame False {
          }
          frame True {
            n831 = local write "Auto Start Temp"(FALSE ("Auto Start Temp")) -> ()
          }
        }
      }
      frame True {
        "Auto stop temp" <- TRUE ("Auto stop temp")
      }
    }
    n832 = local read "Humidity"() -> (w938:bool)
    n833 = case shown="\"HOME\"" w950 {
      frame "HOME" {
        n834 = local write "main tab sub"(enum32{"Page 1", "Page 2"}."Page 1" ("main tab sub")) -> ()
      }
      frame Default {
        n835 = local write "main tab sub"(enum32{"Page 1", "Page 2"}."Page 2" ("main tab sub")) -> ()
      }
    }
    n836 = case shown="True" w949 {
      selector: w949 -> [_ w1285]
      frame False {
      }
      frame True {
        n837 = Not(x=w1285) -> (.not. x?=w1284:bool)
        n838 = local write "Sign In"(w1284) -> ()
        n839 = local write "Main Dashboard Buttons"(T1."Test Setup" ("Main Dashboard Buttons")) -> ()
      }
    }
    n840 = case shown="\"Numeric Display\", Default" "Num/Graph" {
      frame "Numeric Display", Default {
        n841 = property on="Single/Multiple" class="RadioBtnsControl (strict)"("Visible"=FALSE) -> ()  [unwired: 2 in, 2 out]
        n842 = property on="Single - Graph" class="Ring (strict)"("Visible"=FALSE) -> ()  [unwired: 2 in, 2 out]
        n843 = local write "Main Tab Display"(T4."Dashboard 1" ("Main Tab Display")) -> ()
      }
      frame "Graph Display" {
        n844 = property on="Single/Multiple" class="RadioBtnsControl (strict)"("Visible"=TRUE) -> ()  [unwired: 2 in, 2 out]
        n845 = case shown="\"Multiple\"" "Single/Multiple" {
          frame "Single ", Default {
            n846 = property on="Single - Graph" class="Ring (strict)"("Visible"=TRUE) -> ()  [unwired: 2 in, 2 out]
            n847 = local write "Main Tab Display"(T4."Dashboard 3" ("Main Tab Display")) -> ()
          }
          frame "Multiple" {
            n848 = property on="Single - Graph" class="Ring (strict)"("Visible"=FALSE) -> ()  [unwired: 2 in, 2 out]
            n849 = local write "Main Tab Display"(T4."Dashboard 2" ("Main Tab Display")) -> ()
          }
        }
      }
    }
    n850 = local read "Stroke"() -> (w937:bool)
    n851 = local read "USERNAME"() -> (w943:string)
    n852 = local read "USER ID"() -> (w942:string)
    n853 = case shown="True" w940 {
      selector: w940 -> [_ w1220]
      frame False {
      }
      frame True {
        n854 = Not(x=w1220) -> (.not. x?=w1219:bool)
        n855 = local write "Coefficient Of Friction"(w1219) -> ()
        n856 = local write "Tab Control 2"(T6."Coefficient Of Friction" ("Tab Control 2")) -> ()
      }
    }
    n857 = case shown="True" w939 {
      selector: w939 -> [_ w1217]
      frame False {
      }
      frame True {
        n858 = Not(x=w1217) -> (.not. x?=w1215:bool)
        n859 = local write "Air Temperature"(w1215) -> ()
        n860 = local write "Tab Control 2"(T6."Air Temperature" ("Tab Control 2")) -> ()
      }
    }
    n861 = local write "Operator ID"(w942) -> ()
    n862 = case shown="True" w937 {
      selector: w937 -> [_ w1211]
      frame False {
      }
      frame True {
        n863 = Not(x=w1211) -> (.not. x?=w1209:bool)
        n864 = local write "Stroke"(w1209) -> ()
        n865 = local write "Tab Control 2"(T6."Stroke" ("Tab Control 2")) -> ()
      }
    }
    n866 = local write "tested by"(w943) -> ()
    n867 = case shown="True" w938 {
      selector: w938 -> [_ w1214]
      frame False {
      }
      frame True {
        n868 = Not(x=w1214) -> (.not. x?=w1212:bool)
        n869 = local write "Humidity"(w1212) -> ()
        n870 = local write "Tab Control 2"(T6."Humidity" ("Tab Control 2")) -> ()
      }
    }
    n871 = case shown="\"Advance\"" "Main Dashboard Buttons" {
      tunnel: [T2."HOME" ("Main Tab") T2."Test Setup" ("Main Tab") T2."Acquire" ("Main Tab") T2."Adv Scar" ("Main Tab") T2."Adv Scar Report" ("Main Tab") T2."Compare Files" ("Main Tab") T2."About" ("Main Tab") T2."Advance" ("Main Tab")] -> w947
      frame "Home", Default {
      }
      frame "Test Setup" {
      }
      frame "Dashboard" {
      }
      frame "Imaging" {
      }
      frame "Report" {
      }
      frame "Analysis" {
      }
      frame "About" {
      }
      frame "Advance" {
      }
    }
    n872 = Wait (ms)(milliseconds to wait=u32 100) -> ()  [unwired: 1 out]
    n873 = local read "Main Tab Display"() -> (w941:T4)
    n874 = local write "Main Tab"(w947) -> ()
    n875 = case shown="\"Dashboard 3\"" w941 {
      frame "Dashboard 1", Default {
        n876 = property on="Reset Graph" class="Bool (strict)"("Visible"=FALSE) -> ()  [unwired: 2 in, 2 out]
      }
      frame "Dashboard 2" {
        n877 = property on="Reset Graph" class="Bool (strict)"("Visible"=TRUE) -> ()  [unwired: 2 in, 2 out]
      }
      frame "Dashboard 3" {
        n878 = property on="Reset Graph" class="Bool (strict)"("Visible"=TRUE) -> ()  [unwired: 2 in, 2 out]
      }
    }
    n879 = local read "SCAR MEASURMENT"() -> (w929:enum32{"Auto Scar", "Manual Scar"})
    n880 = local read "Humidity"() -> (w944:bool)
    n881 = local read "Cap Live Image"() -> (w926:bool)
    n882 = local read "Sample Temperature"() -> (w936:bool)
    n883 = local read "Air Temp vs Humidity"() -> (w934:bool)
    n884 = local read "Frequency"() -> (w935:bool)
    n885 = case shown="False" w944 {
      frame False {
        n886 = local write "Humidity On Command"(TRUE ("Humidity On Command")) -> ()
        n887 = case shown="True" "Humidity Off Command" {
          selector: "Humidity Off Command" -> [_ w1227]
          frame False {
          }
          frame True {
            n888 = stacked-sequence {
              frame #0 {
                n889 = local read "WriteHumidity"() -> (w1229:string[])
                n890 = Insert Into Array(array=w1229, new element="R;1" ("new element/subarray")) -> (w1230:string[])  [unwired: 1 in]
                n891 = local write "WriteHumidity"(w1230) -> ()
              }
              frame #1 {
                n892 = Wait (ms)(milliseconds to wait=u32 2000) -> ()  [unwired: 1 out]
              }
              frame #2 {
                n893 = local read "EVENT LOG"() -> (w1236:string)
                n894 = local read "WriteHumidity"() -> (w1233:string[])
                n895 = call "Event Log.vi"("Content"="Humidity Control Off" ("string"), "EVENT LOG"=w1236) -> ("EVENT LOG"=w1237:string)  [unwired: 8 in, 1 out]
                n896 = local write "EVENT LOG"(w1237) -> ()
                n897 = Insert Into Array(array=w1233, new element="R;1" ("new element/subarray")) -> (w1234:string[])  [unwired: 1 in]
                n898 = local write "WriteHumidity"(w1234) -> ()
              }
            }
            n899 = Not(x=w1227) -> (.not. x?=w1226:bool)
            n900 = local write "Humidity Off Command"(w1226) -> ()
          }
        }
      }
      frame True {
        n901 = local write "Humidity Off Command"(TRUE ("Humidity Off Command")) -> ()
        n902 = case shown="False" "Humidity On Command" {
          selector: "Humidity On Command" -> [_ w1241]
          frame False {
          }
          frame True {
            n903 = stacked-sequence {
              frame #0 {
                n904 = local read "Set Rh"() -> (w1247:dbl)
                n905 = Number To Fractional String(number=w1247, precision (6)=i16 2) -> (F-format string=w1248:string)  [unwired: 2 in]
                n906 = local read "WriteHumidity"() -> (w1245:string[])
                n907 = Concatenate Strings("M;" ("new element/subarray"), w1248) -> (w1246:string)
                n908 = Insert Into Array(array=w1245, new element=w1246) -> (w1244:string[])  [unwired: 1 in]
                n909 = local write "WriteHumidity"(w1244) -> ()
              }
              frame #1 {
                n910 = Wait (ms)(milliseconds to wait=u32 1500) -> ()  [unwired: 1 out]
              }
              frame #2 {
                (unwired) "% RH" ("string")
                (unwired) i16 2 ("precision (6)")
                (unwired) "M;" ("new element/subarray")
                n911 = local read "Set Rh"() -> (w1255:dbl)
                n912 = Number To Fractional String(number=w1255, precision (6)=i16 2) -> (F-format string=w1252:string)  [unwired: 2 in]
                n913 = local read "WriteHumidity"() -> (w1257:string[])
                n914 = Concatenate Strings("M;" ("new element/subarray"), w1252) -> (w1256:string)
                n915 = Concatenate Strings("Humidity Set to : " ("string"), w1252, "% RH" ("string")) -> (w1250:string)
                n916 = Insert Into Array(array=w1257, new element=w1256) -> (w1258:string[])  [unwired: 1 in]
                n917 = disable-structure shown="Enabled" {
                  frame Enabled {
                    n918 = local read "EVENT LOG"() -> (w1261:string)
                    n919 = call "Event Log.vi"("Content"="Humidity Control On", "EVENT LOG"=w1261) -> ("EVENT LOG"=w1262:string)  [unwired: 8 in, 1 out]
                    n920 = local write "EVENT LOG"(w1262) -> ()
                  }
                  frame Disabled {
                  }
                }
                n921 = disable-structure shown="Enabled" {
                  disable-tunnel: w1250 -> [_ _]
                  frame Enabled {
                    n922 = local read "EVENT LOG"() -> (w1264:string)
                    n923 = call "Event Log.vi"("Content"="Humidity Control On", "EVENT LOG"=w1264) -> ("EVENT LOG"=w1265:string)  [unwired: 8 in, 1 out]
                    n924 = local write "EVENT LOG"(w1265) -> ()
                  }
                  frame Disabled {
                  }
                }
                n925 = local write "WriteHumidity"(w1258) -> ()
              }
            }
            n926 = Not(x=w1241) -> (.not. x?=w1240:bool)
            n927 = local write "Humidity On Command"(w1240) -> ()
          }
        }
      }
    }
    n928 = Equal?(x=w929, y=enum32{"Auto Scar", "Manual Scar"}."Auto Scar" ("SCAR MEASURMENT")) -> (x = y?=w925:bool)
    n929 = local read "TEST STANDARD"() -> (w932:T3)
    n930 = And(x=w926, y=w925) -> (x .and. y?=w927:bool)
    n931 = case shown="True" w927 {
      selector: w927 -> [_ w1026]
      tunnel: errorcluster {"status"=FALSE, "code"=0, "source"=""} ("error in (no error) 3") -> [_ w1027]
      frame False {
      }
      frame True {
        n932 = stacked-sequence {
          tunnel: w1027 -> [_ _ _ _ _ _ _ w1075]
          tunnel: w1026 -> [_ _ _ _ _ w1056 _ _]
          frame #0 {
            n933 = call "CAMERA LIVE FEED FGV.vi"("Enum - Menu"=CAMERA_LIVE_FEED_ENUM."CAMERA MINIMIZE") -> ()  [unwired: 9 in, 2 out]
          }
          frame #1 {
            n934 = property on="Auto Scar Check  2" class="Clust (strict)"("Visible"=TRUE) -> ()  [unwired: 2 in, 2 out]
          }
          frame #2 {
            n935 = String To Path(string="C:\\LAB-IQ\\Image Calibrate v01.dcf") -> (path=w1032:path)
            n936 = Open/Create/Replace File ("Open File")(file path (use dialog)=w1032) -> (refnum out=w1033:refnum<file>)  [unwired: 5 in, 2 out]
            n937 = for {
              N: 4 -> [_]
              tunnel: w1033 -> [w1039]
              i -> [w1035]
              n938 = Read from Text File ("Read File")(file (use dialog)=w1039) -> (text=w1040:string)  [unwired: 3 in, 3 out]
              n939 = String Subset(string=w1040, offset (0)=6, length (rest)=10 ("length (rest)")) -> (substring=w1036:string)
              n940 = Fract/Exp String To Number(string=w1036) -> (number=w1034:dbl)  [unwired: 3 in, 1 out]
              n941 = case shown="0" w1035 {
                tunnel: w1034 -> [w1041 w1042 _ w1043 _]
                frame 0 {
                  "5x Gain" <- w1041
                }
                frame 1 {
                  "10x Gain" <- w1042
                }
                frame 2 {
                }
                frame 3 {
                  "100x gain" <- w1043
                }
                frame 4, Default {
                }
              }
            }
          }
          frame #3 {
            n942 = local read "FILE 3"() -> (w1049:string)
            n943 = call <vilib>:"Trim Whitespace.vi"("string"="C:\\LAB-IQ\\images\\") -> ("trimmed string"=w1051:string)  [unwired: 1 in]
            n944 = String To Path(string=w1051) -> (path=w1050:path)
            n945 = Concatenate Strings(w1049, ".png" ("string")) -> (w1048:string)
            n946 = Build Path(base path=w1050, name or relative path=w1048) -> (appended path=w1046:path)
            "Image path" <- w1046
            n947 = Path To String(path=w1046) -> (string=w1045:string)
            n948 = call "CAMERA LIVE FEED FGV.vi"("Enum - Menu"=CAMERA_LIVE_FEED_ENUM."CAMERA SAVE", "Image Path"=w1045) -> ()  [unwired: 8 in, 2 out]
          }
          frame #4 {
            n949 = One Button Dialog(message="Image saved successfully") -> ()  [unwired: 1 in, 1 out]
          }
          frame #5 {
            n950 = local read "TEST STANDARD"() -> (w1055:T3)
            n951 = local read "Magnification len live scar"() -> (w1067:string)
            n952 = Not(x=w1056) -> (.not. x?=w1057:bool)
            n953 = local write "Cap Live Image"(w1057) -> ()
            n954 = case shown="\"ISO 12156\"" w1055 {
              tunnel: ["ASTM D6079" "ISO 12156"] -> w1054
              frame "ASTM D6079", Default {
              }
              frame "ISO 12156" {
              }
            }
            n955 = case shown="\"5x\", Default" w1067 {
              tunnel: [w1070 w1071] -> w1066
              frame "5x", Default {
                n956 = local read "5x Gain"() -> (w1070:dbl)
              }
              frame "10x" {
                # "5x"
                n957 = local read "10x Gain"() -> (w1071:dbl)
              }
            }
            n958 = local read "Image path"() -> (w1065:path)
            n959 = local read "FILE 3"() -> (w1058:string)
            n960 = call "EDGE DETCTION.vi"("GAIN VALUE"=w1066, "Image Path"=w1065) -> ("error out"=w1064:errorcluster, "return value"=w1063:cluster{string, string, dbl, dbl, dbl})  [unwired: 8 in]
            n961 = Bundle By Name(cluster=T20 {"File Name"="", "Test Method"="", "Operator"="", "Fuel Description"="", "Date and time"=""} ("Main Ref"), "File Name"=w1058, "Test Method"=w1054) -> (w1059:T20)
            n962 = call "duf file read.vi"("error in (no error)"=w1064, "Main Ref"=w1059) -> ("error out"=w1062:errorcluster, "Main Ref 2"=w1060:T20)  [unwired: 8 in]
            n963 = call "EDGE DETECTION REPORT.vi"("error in (no error)"=w1062, "return value 2"=w1063, "Main Ref"=w1060) -> ()  [unwired: 8 in, 1 out]
          }
          frame #6 {
            n964 = property on="Auto Scar Check  2" class="Clust (strict)"("Visible"=FALSE) -> ()  [unwired: 2 in, 2 out]
          }
          frame #7 {
            n965 = call "CAMERA LIVE FEED FGV.vi"("Enum - Menu"=CAMERA_LIVE_FEED_ENUM."CAMERA MINIMIZE", "error in (no error)"=w1075) -> ()  [unwired: 8 in, 2 out]
            n966 = local write "Main Dashboard Buttons"(T1."Home" ("Main Dashboard Buttons")) -> ()
            n967 = local write "Main Tab"(T2."HOME" ("Main Tab")) -> ()
          }
        }
      }
    }
    n968 = local read "Heater Button"() -> (w933:bool)
    n969 = case shown="True" w935 {
      selector: w935 -> [_ w1205]
      frame False {
      }
      frame True {
        n970 = Not(x=w1205) -> (.not. x?=w1203:bool)
        n971 = local write "Frequency"(w1203) -> ()
        n972 = local write "Tab Control 2"(T6."Frequency" ("Tab Control 2")) -> ()
      }
    }
    n973 = case shown="True" w934 {
      selector: w934 -> [_ w1202]
      frame False {
      }
      frame True {
        n974 = Not(x=w1202) -> (.not. x?=w1200:bool)
        n975 = local write "Air Temp vs Humidity"(w1200) -> ()
        n976 = local write "Tab Control 2"(T6."Air Temp vs Rh" ("Tab Control 2")) -> ()
      }
    }
    n977 = case shown="True" w936 {
      selector: w936 -> [_ w1208]
      frame False {
      }
      frame True {
        n978 = Not(x=w1208) -> (.not. x?=w1206:bool)
        n979 = local write "Sample Temperature"(w1206) -> ()
        n980 = local write "Tab Control 2"(T6."Sample Temperature" ("Tab Control 2")) -> ()
      }
    }
    n981 = case shown="\"Custom\"" w932 {
      frame "ASTM D6079", Default {
        w1181 = "ASTM D6079 TEST CONDITIONS" ("Standard 2")
        n982 = local write "Standard 2"(w1181) -> ()
        n983 = local write "Standard"(w1181) -> ()
      }
      frame "ISO 12156" {
        w1182 = "ISO 12156 TEST CONDITIONS" ("Standard 2")
        n984 = local write "Standard 2"(w1182) -> ()
        n985 = local write "Standard"(w1182) -> ()
      }
      frame "CEC F-096-A-06" {
        w1183 = "CEC F-096-A-06 TEST CONDITIONS" ("Standard 2")
        n986 = local write "Standard 2"(w1183) -> ()
        n987 = local write "Standard"(w1183) -> ()
      }
      frame "Custom" {
        w1184 = "CUSTOM TEST CONDITIONS" ("Standard 2")
        n988 = local write "Standard 2"(w1184) -> ()
        n989 = local write "Standard"(w1184) -> ()
      }
    }
    n990 = case shown="True" w933 {
      frame False {
        n991 = local write "Temperature On Command"(TRUE ("Temperature On Command")) -> ()
        n992 = case shown="True" "Temperature Off Command" {
          selector: "Temperature Off Command" -> [_ w1188]
          frame False {
          }
          frame True {
            n993 = Not(x=w1188) -> (.not. x?=w1187:bool)
            n994 = local read "EVENT LOG"() -> (w1191:string)
            n995 = local write "Temperature Off Command"(w1187) -> ()
            n996 = call "Event Log.vi"("Content"="Heater Off", "EVENT LOG"=w1191) -> ("EVENT LOG"=w1190:string)  [unwired: 8 in, 1 out]
            n997 = local write "EVENT LOG"(w1190) -> ()
          }
        }
      }
      frame True {
        n998 = local write "Temperature Off Command"(TRUE ("Temperature Off Command")) -> ()
        n999 = case shown="True" "Temperature On Command" {
          selector: "Temperature On Command" -> [_ w1195]
          frame False {
          }
          frame True {
            n1000 = Not(x=w1195) -> (.not. x?=w1194:bool)
            n1001 = local write "Temperature On Command"(w1194) -> ()
            n1002 = disable-structure shown="Enabled" {
              disable-tunnel: "Heater On" -> [w1197 _]
              frame Enabled {
                n1003 = local read "EVENT LOG"() -> (w1198:string)
                n1004 = call "Event Log.vi"("Content"=w1197, "EVENT LOG"=w1198) -> ("EVENT LOG"=w1199:string)  [unwired: 8 in, 1 out]
                n1005 = local write "EVENT LOG"(w1199) -> ()
              }
              frame Disabled {
              }
            }
          }
        }
      }
    }
    n1006 = local read "Main Tab"() -> (w924:T2)
    n1007 = case shown="\"About\"" w924 {
      frame "HOME", Default {
        w970 = T15."Enabled" ("Disabled")
        n1008 = local read "Service Password enable"() -> (w969:bool)
        n1009 = property on="Imaging" class="Bool (strict)"("DisabledEnum"=w970) -> ()  [unwired: 2 in, 2 out]
        n1010 = property on="Dashboard" class="Bool (strict)"("DisabledEnum"=w970) -> ()  [unwired: 2 in, 2 out]
        n1011 = property on="Test Setup" class="Bool (strict)"("DisabledEnum"=w970) -> ()  [unwired: 2 in, 2 out]
